vi "SCLN_GetResponseFromServer.vi"(2 "error in (no error)":errorcluster, 3 "Index for Response":i32) -> (0 "error out":errorcluster, 1 "Message":string)   [LabVIEW 2015]
uses:
  SCLN_RW_Select.ctl
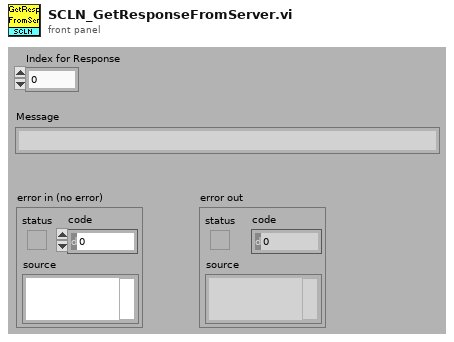
[diagram p1: front panel]
types:
  T1 = typedef "SCLN_RW_Select.ctl" = enum16{"Read", "Write"}
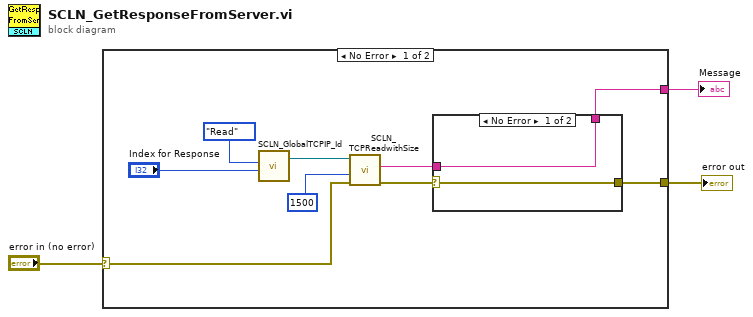
[diagram p0: block diagram]
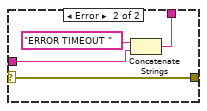
[diagram p2: hidden frame]
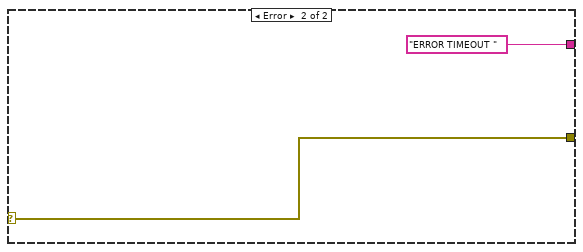
[diagram p3: hidden frame]
diagram:
  n1 = case shown="No Error" "error in (no error)" {
    selector: "error in (no error)" -> [w4 w19]
    tunnel: [w7 "ERROR TIMEOUT "] -> w3
    tunnel: [w5 w19] -> w2
    frame No Error {
      n2 = call "SCLN_GlobalTCPIP_Id.vi"("Element"="Index for Response", "Operation"=SCLN_RW_Select."Read" ("GBL_RW")) -> ("TCPIP_Id Read"=w11:refnum<k5>)  [unwired: 2 in, 1 out]
      n3 = call "SCLN_TCPReadwithSize.vi"("error in (no error)"=w4, "timeout ms (600)"=1500, "connection ID"=w11) -> ("error out"=w9:errorcluster, "data out"=w8:string)  [unwired: 6 in, 1 out]
      n4 = case shown="No Error" w9 {
        selector: w9 -> [w13 w15]
        tunnel: [w14 w18] -> w7
        tunnel: w8 -> [w14 w16]
        tunnel: [w13 w15] -> w5
        frame No Error {
        }
        frame Error {
          n5 = Concatenate Strings("ERROR TIMEOUT ", w16) -> (w18:string)
        }
      }
    }
    frame Error {
    }
  }
  "Message" <- w3
  "error out" <- w2
